vi "Synchronize to PPS - cRIO.vi"() -> ()   [LabVIEW 2020]
uses:
  FPGA Timekeeper.lvlib
  <vilib>/platform/TimedLoop/XDataNode/XDataNode.xnode
  <vilib>/Platform/TimedLoop/XDataNode/nitl_modes.ctl
  <vilib>/Platform/TimedLoop/XDataNode/XDNodeRunTimeDep.lvlib
  <vilib>/Platform/TimedLoop/XDataNode/wakeup.ctl
  <vilib>/Platform/TimedLoop/XDataNode/timing_clust.ctl
  <vilib>/eio/EIONode/EIONode.xnode
panel:
  out "offset from time reference":i32
  out "FPGA Timekeeper locked":bool
  out "FPGA Timekeeper time (ns)":u64
  in  "absolute time offset(ns)":u64
  # "This example synchronizes the FPGA Timekeeper on a CompactRIO FPGA target with a pulse per second (PPS)."
  # "FPGA Timekeeper"
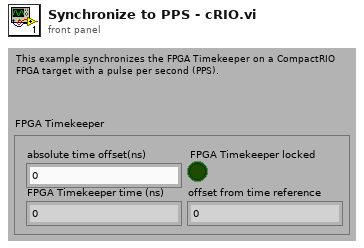
[diagram p1: front panel]
types:
  T1 = typedef "XDNodeRunTimeDep.lvlib/timing_clust.ctl" = cluster{"Expected End [f-1]":u64, "Actual End [f-1]":u64, "Finished Late? [f-1]":bool, "Expected End [i-1]":u64, "Actual End [i-1]":u64, "Finished Late? [i-1]":bool, "Expected Start [i]":u64, "Actual Start [i]":u64, "Expected Start [f]":u64, "Actual Start [f]":u64, "Source Name":string, "Structure Name":string, "Period":i64, "Deadline":i64, "Offset":i64, "Start":i64, "Priority":i32, "Timeout":i32, "Mode":T2, "Wakeup Reason":T3, "Error":errorcluster, "Source Type":string, "Secondary Source Type":string, "Global End Time":u64, "Global Start Time":u64, "Frame Duration":u64, "Iteration Duration":u64, "Assigned CPU":i32, "I/O Scan Engine Mode":u32}
  T2 = typedef "XDNodeRunTimeDep.lvlib/nitl_modes.ctl" = enum32{"No Change", "Process missed periods, maintain original phase", "Discard missed periods, maintain original phase", "Process missed periods, ignore original phase", "Discard missed periods, ignore original phase"}
  T3 = typedef "XDNodeRunTimeDep.lvlib/wakeup.ctl" = enum32{"Normal", "Aborted", "Asynchronous wakeup", "Timing source error", "Timed loop error", "Timeout"}
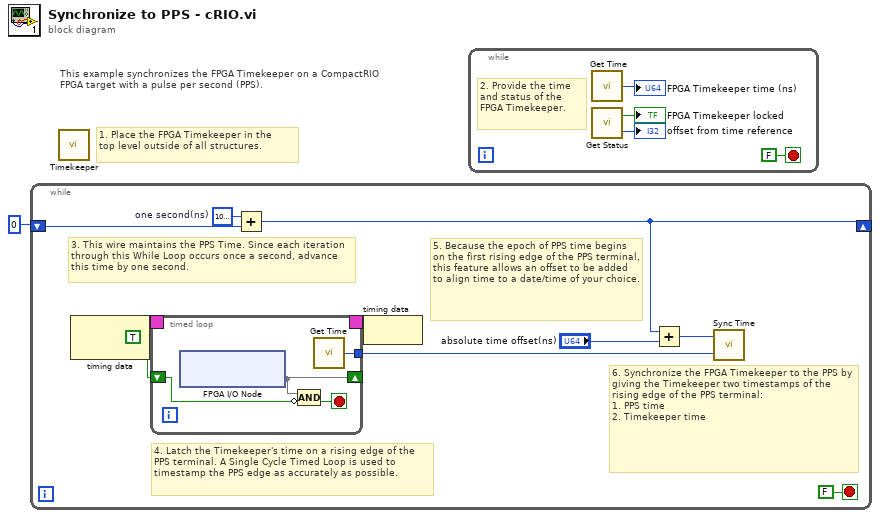
[diagram p0: block diagram]
diagram:
  # "This example synchronizes the FPGA Timekeeper on a CompactRIO FPGA target with a pulse per second (PPS)."
  # "1. Place the FPGA Timekeeper in the\ntop level outside of all structures."
  n1 = while {
    shift-right: [w4] -> _
    shift-left: u64 0 -> [w11]
    stop <- FALSE stop-if-true
    w10 = u64 1000000000  # one second(ns)
    # "5. Because the epoch of PPS time begins on the first rising edge of the PPS terminal, this feature allows an offset to be added to align time to a date/time of your choice."
    # "4. Latch the Timekeeper's time on a rising edge of the PPS terminal. A Single Cycle Timed Loop is used to timestamp the PPS edge as accurately as possible."
    # "3. This wire maintains the PPS Time. Since each iteration through this While Loop occurs once a second, advance this time by one second."
    # "6. Synchronize the FPGA Timekeeper to the PPS by giving the Timekeeper two timestamps of the rising edge of the PPS terminal:\n1. PPS time\n2. Timekeeper time"
    n2 = node-c288() -> (w9:T1)  [unwired: 1 in]
    n3 = timed-loop {
      timing: w9 -> [_]
      timing-out: [_] -> w8
      shift-right: [w12] -> _
      shift-left: TRUE ("Mod1/DIO0") -> [w15]
      tunnel: [w13] -> w6
      stop <- w14 stop-if-true
      n4 = xnode "FPGA I/O Node"() -> ("Mod1/DIO0"=w12)  [unwired: 1 in, 1 out]
      n5 = Compound Arithmetic op=AND(w12, invert w15) -> (w14:bool)
      n6 = call "Get Time.vi"() -> ("time (ns)"=w13:u64)
    }
    n7 = Add(x=w10, y=w11) -> (x+y=w4:u64)
    n8 = node-c288(w8) -> ()
    n9 = Add(x=w4, y="absolute time offset(ns)") -> (x+y=w3:u64)
    n10 = call "Sync Time.vi"("FPGA Timekeeper time (ns)"=w6, "time reference time (ns)"=w3) -> ()
  }
  n11 = call "Timekeeper.vi"() -> ()  [unwired: 12 in]
  n12 = while {
    stop <- FALSE stop-if-true
    # "2. Provide the time\nand status of the\nFPGA Timekeeper."
    n13 = call "Get Time.vi"() -> ("time (ns)"=→"FPGA Timekeeper time (ns)":u64)
    n14 = call "Get Status.vi"() -> ("FPGA Timekeeper locked"=→"FPGA Timekeeper locked":bool, "offset from time reference"=→"offset from time reference":i32)
  }
